vi "Log Data.vi"(7 "Number of Blocks Saved in":i32 caption="保存的数据块数输入", 8 "error in (no error)":errorcluster caption="错误输入（无错误）", 9 "Waveform Data Array":waveform(sgl)[](array[waveform]) caption="波形数组", 10 "Acquisition and Logging Configuration":T1={"Samples per Read"=100, "Number of Reads to Save"=20, "Number of Channels"=4, "Channel Scale Array"=[1.0, 1.0, 1.0, 1.0], "Channel Names"=[], "Trigger - RMS Value"=0.9999999999999994, "Trigger - Channel"=0, "Trigger - Time (Minute)"=10, "TDMS Properties"=[], "Data File Name"="cRIO_Data", "Date Rate"=20} caption="采集与记录配置" {"Date Rate" items=["51.200 kS/s (NI 9234)"=1, "25.600 kS/s (NI 9234)"=2, "17.067 kS/s (NI 9234)"=3, "12.80 kS/s (NI 9234)"=4, "10.240 kS/s (NI 9234)"=5, "8.533 kS/s (NI 9234)"=6, "7.314 kS/s (NI 9234)"=7, "6.400 kS/s (NI 9234)"=8, "5.689 kS/s (NI 9234)"=9, "5.120 kS/s (NI 9234)"=10, "4.654 kS/s (NI 9234)"=11, "4.267 kS/s (NI 9234)"=12, "3.938 kS/s (NI 9234)"=13, "3.657 kS/s (NI 9234)"=14, "3.413 kS/s (NI 9234)"=15, "3.200 kS/s (NI 9234)"=16, "3.012 kS/s (NI 9234)"=17, "2.845 kS/s (NI 9234)"=18, "2.695 kS/s (NI 9234)"=19, "2.560 kS/s (NI 9234)"=20, "2.438 kS/s (NI 9234)"=21, "2.328 kS/s (NI 9234)"=22, "2.226 kS/s (NI 9234)"=23, "2.133 kS/s (NI 9234)"=24, "2.048 kS/s (NI 9234)"=25, "1.969 kS/s (NI 9234)"=26, "1.896 kS/s (NI 9234)"=27, "1.829 kS/s (NI 9234)"=28, "1.765 kS/s (NI 9234)"=29, "1.707 kS/s (NI 9234)"=30, "1.652 kS/s (NI 9234)"=31]}, 11 "TDMS File Reference":refnum<k34> caption="TDMS文件引用") -> (0 "error out":errorcluster caption="错误输出", 3 "Logging Complete?":bool caption="记录完成？", 5 "Number of Blocks Saved out":i32 caption="保存的数据块数输出")   [LabVIEW 2013]
doc: "读取DMA FIFO的波形数据。"
uses:
  controls/Acquisition and Logging Configuration.ctl
  controls/TDMS Properties.ctl
  <vilib>/LabVIEW Targets/FPGA/cRIO/shared/nicrio_ModuleControls/nicrio_cRIO-9234_DataRatesRing2.ctl
  <vilib>/Analysis/5stat.llb/RMS (DBL).vi
  <vilib>/Analysis/NI_AALPro.lvlib
panel:
  # "通道"
  # "保存"
  # "采样"
  # "触发"
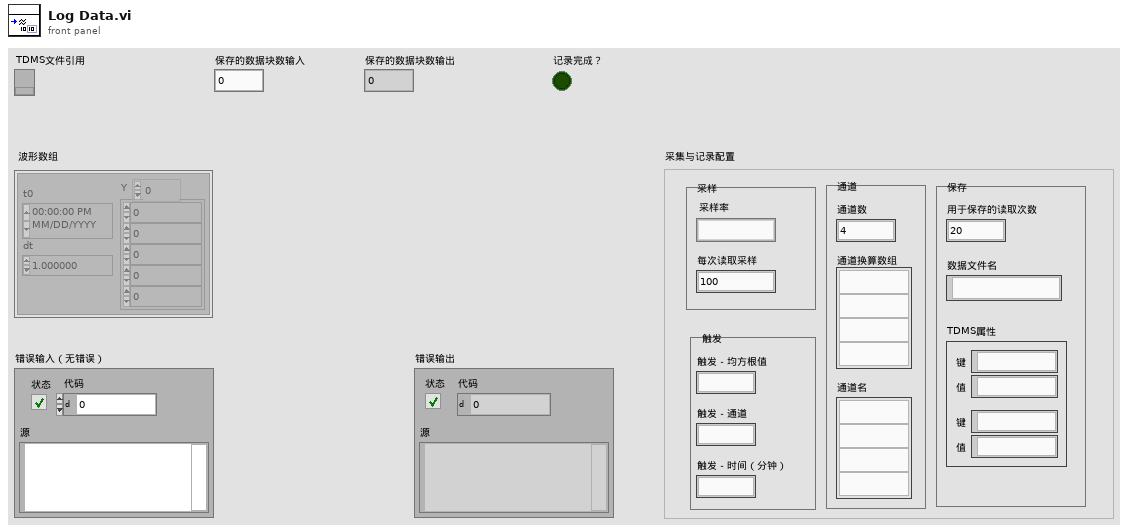
[diagram p1: front panel]
types:
  T1 = typedef "Acquisition and Logging Configuration.ctl" = cluster{"Samples per Read":i32, "Number of Reads to Save":i32, "Number of Channels":i32, "Channel Scale Array":fxp<+,24,12>[], "Channel Names":string[], "Trigger - RMS Value":dbl, "Trigger - Channel":i32, "Trigger - Time (Minute)":i32, "TDMS Properties":T2[], "Data File Name":string, "Date Rate":T3}
  T2 = typedef "TDMS Properties.ctl" = cluster{"Name":string, "Value":string}
  T3 = typedef "nicrio_cRIO-9234_DataRatesRing2.ctl" = u16
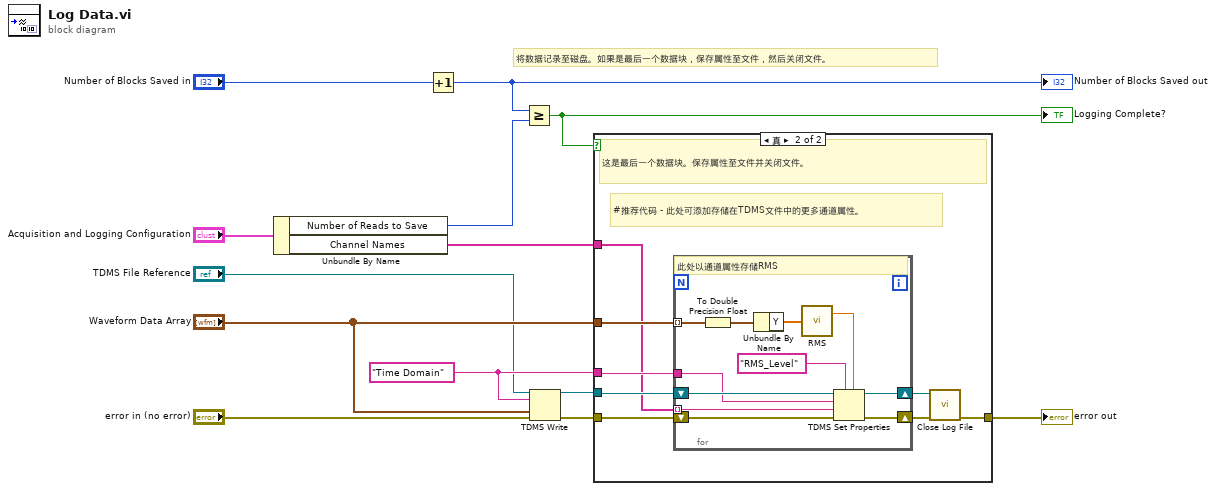
[diagram p0: block diagram]
diagram:
  w7 = "Time Domain" ("group name in (Untitled)")
  # "将数据记录至磁盘。如果是最后一个数据块，保存属性至文件，然后关闭文件。"
  n1 = Unbundle By Name("Acquisition and Logging Configuration") -> ("Number of Reads to Save"=w11:i32, "Channel Names"=w3:string[])
  n2 = Increment(x="Number of Blocks Saved in") -> (x+1=w12:i32)
  "Number of Blocks Saved out" <- w12
  n3 = Greater Or Equal?(x=w12, y=w11) -> (x >= y?=w10:bool)
  "Logging Complete?" <- w10
  n4 = TDMS Write(0:"TDMS File Reference", 5:w7, 9:"Waveform Data Array", 11:"error in (no error)") -> (4:w9:refnum<k34>, 15:w8:errorcluster)  [unwired: 2 in, 2 out]
  n5 = case shown="真" w10 {
    tunnel: w9 -> [_ w20]
    tunnel: w8 -> [w14 w22]
    tunnel: [w14 w16] -> w6
    tunnel: w7 -> [_ w19]
    tunnel: "Waveform Data Array" -> [_ w18]
    tunnel: w3 -> [_ w15]
    frame False {
      # "不要关闭文件。这不是最后一个数据块。"
    }
    frame True {
      # "#推荐代码 - 此处可添加存储在TDMS文件中的更多通道属性。"
      # "这是最后一个数据块。保存属性至文件并关闭文件。"
      n6 = for {
        tunnel: w19 -> [w30]
        shift-right: [w32] -> w21
        shift-left: w22 -> [w31]
        tunnel: w15 -> [w29] mode=indexing
        tunnel: w18 -> [w27] mode=indexing
        shift-right: [w24] -> w17
        shift-left: w20 -> [w33]
        # "此处以通道属性存储RMS"
        n7 = To Double Precision Float(number=w27) -> (double precision float=w28:waveform(dbl))
        n8 = Unbundle By Name(w28) -> ("Y"=w23:dbl[])
        n9 = call-poly <vilib>:"RMS.vi"("X"=w23) -> ("rms value"=w26:dbl)  [unwired: 1 out]
        n10 = TDMS Set Properties(5:w26, 7:"RMS_Level" ("property names"), 8:w31, 9:w29, 10:w30, 11:w33) -> (0:w32:errorcluster, 3:w24:refnum<k34>)  [unwired: 2 out]
      }
      n11 = call "Close Log File.vi"("error in (no error)"=w21, "Log File"=w17) -> ("error out"=w16:errorcluster)  [unwired: 9 in]
    }
  }
  "error out" <- w6
